vi "Update ROI.vi"(11 "Detail Graph in":refnum<class "Graph with Section Views.lvclass">) -> (3 "Detail Graph out":refnum<class "Graph with Section Views.lvclass">)   [LabVIEW 2023, in "Graph with Section Views.lvclass"]
uses:
  Graph with Section Views.lvclass
  Graph with Section Views.lvclass/Graph with Section Views.ctl
  Base Graph/Base Graph.lvclass
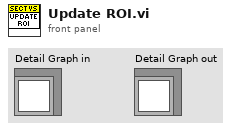
[diagram p1: front panel]
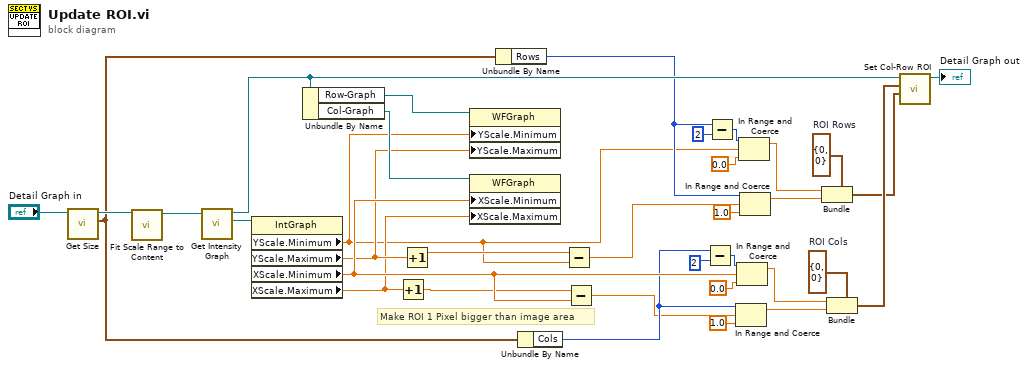
[diagram p0: block diagram]
diagram:
  w1 = cluster{"Index":u32, "Length":u32} {"Index"=0, "Length"=0}  # ROI Rows
  w4 = cluster{"Index":u32, "Length":u32} {"Index"=0, "Length"=0}  # ROI Cols
  # "Make ROI 1 Pixel bigger than image area"
  n1 = call "Get Size.vi"("Base Graph in"="Detail Graph in") -> ("Size"=w21:cluster{"Rows":u32, "Cols":u32}, "Base Graph out"=w25:refnum<class "Graph with Section Views.lvclass">)  [unwired: 9 in]
  n2 = call "Fit Scale Range to Content.vi"("Base Graph in"=w25) -> ("Base Graph out"=w28:refnum<class "Graph with Section Views.lvclass">)  [unwired: 10 in]
  n3 = call "Get Intensity Graph.vi"("Base Graph in"=w28) -> ("Intensity Graph"=w33:refnum<vi>, "Base Graph out"=w32:refnum<class "Graph with Section Views.lvclass">)  [unwired: 9 in]
  n4 = property on="Property Node" class="IntGraph"(reference=w33) -> ("YScale.Minimum"=w5:dbl, "YScale.Maximum"=w27:dbl, "XScale.Minimum"=w29:dbl, "XScale.Maximum"=w26:dbl)  [unwired: 1 in, 2 out]
  n5 = Unbundle By Name(w32) -> ("Row-Graph"=w31:refnum<vi>, "Col-Graph"=w30:refnum<vi>)
  n6 = Increment(x=w26) -> (x+1=w24:dbl)
  n7 = Increment(x=w27) -> (x+1=w23:dbl)
  n8 = property on="Property Node" class="WFGraph"(reference=w31, "YScale.Minimum"=w5, "YScale.Maximum"=w27) -> ()  [unwired: 1 in, 2 out]
  n9 = property on="Property Node" class="WFGraph"(reference=w30, "XScale.Minimum"=w29, "XScale.Maximum"=w26) -> ()  [unwired: 1 in, 2 out]
  n10 = Unbundle By Name(w21) -> ("Rows"=w9:u32)
  n11 = Unbundle By Name(w21) -> ("Cols"=w20:u32)
  n12 = Subtract(x=w23, y=w5) -> (x-y=w7:dbl)
  n13 = Subtract(x=w24, y=w29) -> (x-y=w12:dbl)
  n14 = Subtract(x=w20, y=u32 2) -> (x-y=w10:u32)
  n15 = Subtract(x=w9, y=u32 2) -> (x-y=w11:u32)
  n16 = In Range and Coerce(upper limit=w20, x=w12, lower limit=1.0) -> (coerced(x)=w14:dbl)  [unwired: 1 out]
  n17 = In Range and Coerce(upper limit=w10, x=w29, lower limit=0.0) -> (coerced(x)=w19:dbl)  [unwired: 1 out]
  n18 = In Range and Coerce(upper limit=w11, x=w5, lower limit=0.0) -> (coerced(x)=w22:dbl)  [unwired: 1 out]
  n19 = In Range and Coerce(upper limit=w9, x=w7, lower limit=1.0) -> (coerced(x)=w15:dbl)  [unwired: 1 out]
  n20 = Bundle(cluster=w1, "Index"=w22, "Length"=w15) -> (w2:cluster{"Index":u32, "Length":u32})
  n21 = Bundle(cluster=w4, "Index"=w19, "Length"=w14) -> (w3:cluster{"Index":u32, "Length":u32})
  n22 = call "Set Col-Row ROI.vi"("ROI Rows"=w2, "ROI Cols"=w3, "Base Graph in"=w32) -> ("Base Graph out"=→"Detail Graph out":refnum<class "Graph with Section Views.lvclass">)  [unwired: 8 in]
